vi "Pre Build Icon Editor PPL.vi"(6 "Top Level/Always Included VIs":path[](array[path]), 7 "Main Destination Path":path, 9 "Target Name":string, 10 "Build Specification Name":string, 11 "Project Path":path) -> (0 "error out":errorcluster)   [LabVIEW 2012]
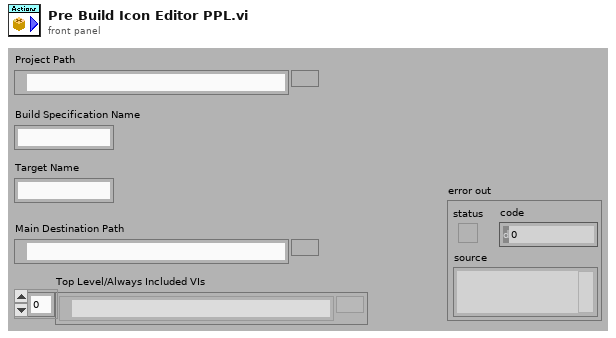
[diagram p1: front panel]
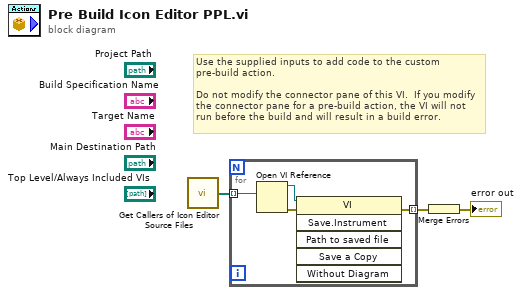
[diagram p0: block diagram]
diagram:
  # "Use the supplied inputs to add code to the custom pre-build action.\n\nDo not modify the connector pane of this VI.  If you modify the connector pane for a pre-build action, the VI will not run before the build and will result in a build error."
  n1 = call <resource>:"Get Callers of Icon Editor Source Files.vi"() -> ("CallersOfIconEditorSourceFiles"=w1:path[])  [unwired: 1 in]
  n2 = for {
    tunnel: w1 -> [w7] mode=indexing
    tunnel: [w4] -> w2 mode=indexing
    n3 = Open VI Reference(vi path=w7) -> (vi reference=w6:refnum<vi>, error out=w5:errorcluster)  [unwired: 5 in]
    n4 = invoke class="VI" method="Save.Instrument"(reference=w6, error in=w5) -> (error out=w4:errorcluster)  [unwired: 4 in, 5 out]
  }
  n5 = Merge Errors(w2) -> (→"error out":errorcluster)
